vi "Lin_Rohner_lab2B_question5.vi"() -> ()   [LabVIEW 2019]
uses:
  <vilib>/Platform/TimedLoop/XDataNode/timing_clust.ctl
  <vilib>/Platform/TimedLoop/XDataNode/nitl_modes.ctl
  <vilib>/Platform/TimedLoop/XDataNode/wakeup.ctl
  <vilib>/Analysis/3filter.llb/Filter Passband Type.ctl
  <vilib>/DAQmx/write.llb/DAQmx Write (Analog DBL 1Chan 1Samp).vi
  <vilib>/DAQmx/read.llb/DAQmx Read (Analog DBL 1Chan 1Samp).vi
  <vilib>/DAQmx/create/channels.llb/DAQmx Create Channel (AO-Voltage-Basic).vi
  <vilib>/DAQmx/miscellaneous.llb/DAQmx Fill In Error Info.vi
  <vilib>/DAQmx/create/channels.llb/DAQmx Create Channel (AI-Voltage-Basic).vi
  <vilib>/platform/TimedLoop/XDataNode/XDataNode.xnode
  <vilib>/Platform/TimedLoop/XDataNode/XDNodeRunTimeDep.lvlib
  <vilib>/Analysis/NI_AALBase.lvlib
  <vilib>/ptbypt/NI_PtbyPt.lvlib
panel:
  out "Current through Shunt":dbl(graph)
  in  "low cutoff freq for the differential voltage measurement at Shunt":dbl=0.12500000000000006 format="%0.4f"
  out "Motor Control Voltage":dbl(graph)
  in  "stop":bool
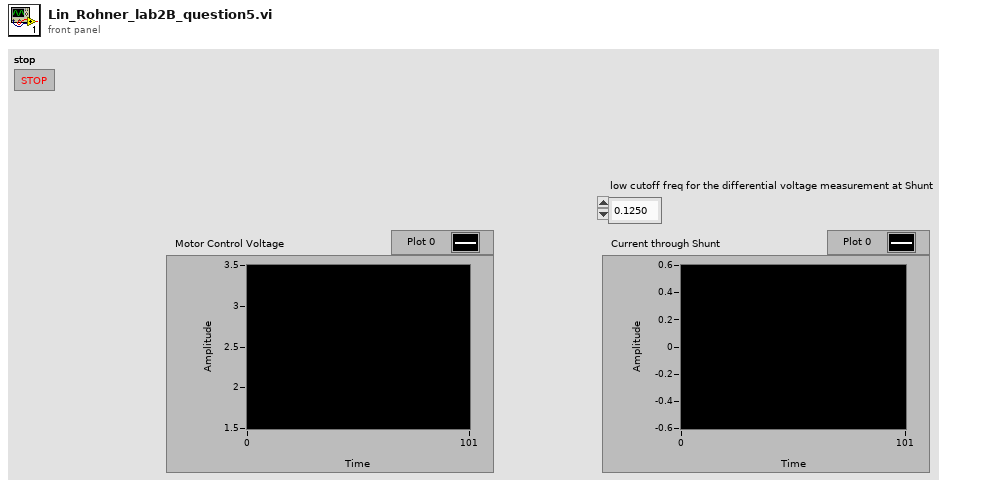
[diagram p1: front panel]
types:
  T1 = typedef "NI_AALBase.lvlib/Filter Passband Type.ctl" = enum32{"Lowpass", "Highpass", "Bandpass", "Bandstop"}
  T2 = typedef "XDNodeRunTimeDep.lvlib/timing_clust.ctl" = cluster{"Expected End [f-1]":u64, "Actual End [f-1]":u64, "Finished Late? [f-1]":bool, "Expected End [i-1]":u64, "Actual End [i-1]":u64, "Finished Late? [i-1]":bool, "Expected Start [i]":u64, "Actual Start [i]":u64, "Expected Start [f]":u64, "Actual Start [f]":u64, "Source Name":string, "Structure Name":string, "Period":i64, "Deadline":i64, "Offset":i64, "Start":i64, "Priority":i32, "Timeout":i32, "Mode":T3, "Wakeup Reason":T4, "Error":errorcluster, "Source Type":string, "Secondary Source Type":string, "Global End Time":u64, "Global Start Time":u64, "Frame Duration":u64, "Iteration Duration":u64, "Assigned CPU":i32, "I/O Scan Engine Mode":u32}
  T3 = typedef "XDNodeRunTimeDep.lvlib/nitl_modes.ctl" = enum32{"No Change", "Process missed periods, maintain original phase", "Discard missed periods, maintain original phase", "Process missed periods, ignore original phase", "Discard missed periods, ignore original phase"}
  T4 = typedef "XDNodeRunTimeDep.lvlib/wakeup.ctl" = enum32{"Normal", "Aborted", "Asynchronous wakeup", "Timing source error", "Timed loop error", "Timeout"}
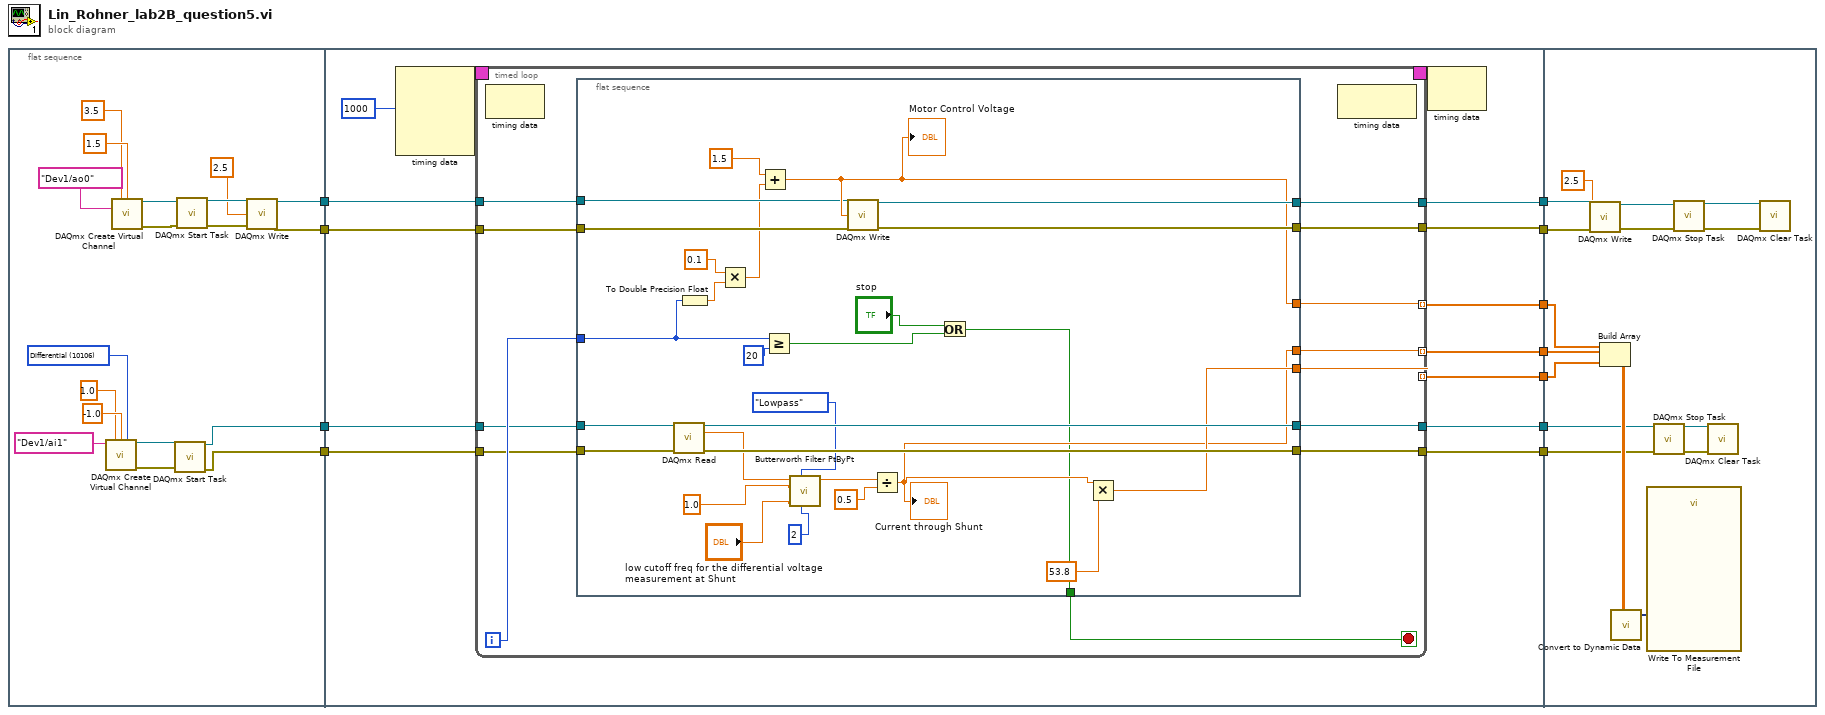
[diagram p0: block diagram]
diagram:
  n1 = flat-sequence {
    tunnel: [w27] -> w4
    tunnel: [w26] -> w3
    tunnel: [w14] -> w2
    tunnel: [w13] -> w1
    tunnel: [w41] -> w11
    tunnel: [w40] -> w10
    tunnel: [w36] -> w9
    tunnel: [w35] -> w8
    tunnel: [w34] -> w7
    tunnel: [w33] -> w6
    tunnel: [w32] -> w5
    tunnel: w4 -> [w31]
    tunnel: w3 -> [w30]
    tunnel: w2 -> [w39]
    tunnel: w1 -> [w38]
    tunnel: w11 -> [w106]
    tunnel: w10 -> [w101]
    tunnel: w9 -> [w97]
    tunnel: w8 -> [w94]
    tunnel: w7 -> [w93]
    tunnel: w6 -> [w92]
    tunnel: w5 -> [w91]
    frame #0 {
      w12 = 10106 items=["Default"=-1, "RSE"=10083, "NRSE"=10078, "Differential"=10106, "Pseudodifferential"=12529] ("input terminal configuration")
      n2 = call-poly <vilib>:"DAQmx Create Virtual Channel.vi"("maximum value"=1.0, "minimum value"=-1.0, "input terminal configuration"=w12, "physical channels"=tag "Dev1/ai1") -> ("task out"=w19:refnum<k21>, "error out"=w18:errorcluster)  [unwired: 10 in]
      n3 = call-poly <vilib>:"DAQmx Create Virtual Channel.vi"("maximum value"=3.5, "minimum value"=1.5, "physical channels"=tag "Dev1/ao0") -> ("task out"=w29:refnum<k21>, "error out"=w25:errorcluster)  [unwired: 11 in]
      n4 = call <vilib>:"DAQmx Start Task.vi"("task/channels in"=w19, "error in"=w18) -> ("task out"=w14:refnum<k21>, "error out"=w13:errorcluster)  [unwired: 12 in]
      n5 = call <vilib>:"DAQmx Start Task.vi"("task/channels in"=w29, "error in"=w25) -> ("task out"=w28:refnum<k21>, "error out"=w24:errorcluster)  [unwired: 12 in]
      n6 = call-poly <vilib>:"DAQmx Write.vi"("task/channels in"=w28, "data"=2.5, "error in"=w24) -> ("task out"=w27:refnum<k21>, "error out"=w26:errorcluster)  [unwired: 10 in, 1 out]
    }
    frame #1 {
      n7 = node-c288(i64 1000 ("Period")) -> (w43:T2)  [unwired: 3 in]
      n8 = timed-loop {
        timing: w43 -> [_]
        timing-out: [_] -> w42
        tunnel: w31 -> [w56]
        tunnel: w30 -> [w54]
        tunnel: [w55] -> w41
        tunnel: [w53] -> w40
        tunnel: w39 -> [w49]
        tunnel: w38 -> [w48]
        tunnel: [w50] -> w36 mode=indexing
        tunnel: [w47] -> w35
        tunnel: [w46] -> w34
        tunnel: [w45] -> w33 mode=indexing
        tunnel: [w44] -> w32 mode=indexing
        i -> [w51]
        stop <- w52 stop-if-true
        n9 = node-c288() -> ()  [unwired: 1 in, 1 out]
        n10 = flat-sequence {
          tunnel: [w78] -> w44
          tunnel: [w79] -> w45
          tunnel: [w80] -> w46
          tunnel: [w81] -> w47
          tunnel: [w82] -> w50
          tunnel: [w83] -> w53
          tunnel: [w84] -> w55
          tunnel: w48 -> [w68]
          tunnel: w49 -> [w69]
          tunnel: w51 -> [w57]
          tunnel: [w59] -> w52
          tunnel: w54 -> [w66]
          tunnel: w56 -> [w67]
          frame #0 {
            n11 = call-poly <vilib>:"DAQmx Read.vi"("task/channels in"=w69, "error in"=w68) -> ("task out"=w81:refnum<k21>, "data"=w71:dbl, "error out"=w80:errorcluster)  [unwired: 11 in]
            n12 = To Double Precision Float(number=w57) -> (double precision float=w58:dbl)
            n13 = Multiply(x=0.1, y=w58) -> (x*y=w64:dbl)
            n14 = Add(x=1.5, y=w64) -> (x+y=w82:dbl)
            "Motor Control Voltage" <- w82
            n15 = Greater Or Equal?(x=w57, y=20 ("x")) -> (x >= y?=w60:bool)
            n16 = call <vilib>:"Butterworth Filter PtByPt.vi"("order"=2, "filter type"=Filter_Passband_Type."Lowpass", "low cutoff freq: fl"="low cutoff freq for the differential voltage measurement at Shunt", "sampling freq: fs"=1.0, "x"=w71) -> ("Filtered x"=w75:dbl)  [unwired: 4 in, 1 out]
            n17 = call-poly <vilib>:"DAQmx Write.vi"("task/channels in"=w67, "data"=w82, "error in"=w66) -> ("task out"=w84:refnum<k21>, "error out"=w83:errorcluster)  [unwired: 10 in, 1 out]
            n18 = Divide(x=w75, y=0.5) -> (x/y=w78:dbl)
            "Current through Shunt" <- w78
            n19 = Or(x="stop", y=w60) -> (x .or. y?=w59:bool)
            n20 = Multiply(x=w78, y=53.8) -> (x*y=w79:dbl)
          }
        }
        n21 = node-c288() -> ()  [unwired: 1 in, 1 out]
      }
      n22 = node-c288(w42) -> ()  [unwired: 1 out]
    }
    frame #2 {
      n23 = call-poly <vilib>:"DAQmx Write.vi"("task/channels in"=w106, "data"=2.5, "error in"=w101) -> ("task out"=w105:refnum<k21>, "error out"=w102:errorcluster)  [unwired: 10 in, 1 out]
      n24 = Build Array(w97, w91, w92) -> (w96:dbl[][])
      n25 = call "Convert to Dynamic Data"("2D Array"=w96) -> ("Dynamic Data Type"=w95:dynamicdata)  [unwired: 3 in]
      n26 = call "Write To Measurement File"("Signals"=w95) -> ()  [unwired: 16 in, 3 out]
      n27 = call <vilib>:"DAQmx Stop Task.vi"("task/channels in"=w94, "error in"=w93) -> ("task out"=w99:refnum<k21>, "error out"=w98:errorcluster)  [unwired: 12 in]
      n28 = call <vilib>:"DAQmx Stop Task.vi"("task/channels in"=w105, "error in"=w102) -> ("task out"=w104:refnum<k21>, "error out"=w103:errorcluster)  [unwired: 12 in]
      n29 = call <vilib>:"DAQmx Clear Task.vi"("task in"=w99, "error in"=w98) -> ()  [unwired: 13 in, 1 out]
      n30 = call <vilib>:"DAQmx Clear Task.vi"("task in"=w104, "error in"=w103) -> ()  [unwired: 13 in, 1 out]
    }
  }
